vi "ConnectionClosed.vi"(6 "FinaErrorCode":i32, 8 "error in (no error)":errorcluster, 9 "ClientIP":string, 10 "ConnectionNumber":i32, 11 "TCP_Server in":refnum<class "TCP_Server.lvclass">) -> (0 "error out":errorcluster, 3 "TCP_Server out":refnum<class "TCP_Server.lvclass">)   [LabVIEW 2023, in "TCP_Server.lvlib" / "TCP_Server.lvclass"]
uses:
  TCP_Server.lvclass
  TCP_Server.lvclass/TCP_Server.ctl
  <vilib>/ActorFramework/Stop Msg/Stop Msg.lvclass
  76787049-4297-4f56-aecd-24274861dc6b.vi
  <vilib>/ActorFramework/Message Enqueuer/Message Enqueuer.lvclass
  TCP_Listener/TypeDefinitions/ConnectionInformation.ctl
  TCP_Listener/TCP_Listener.lvlib
  TypeDeclarations/ServerConnection.ctl
  TCP_Server.lvlib
  TCP_serverGUI/TCP_serverGUI Messages/UpdateConnectionsListbox Msg/UpdateConnectionsListbox Msg.lvclass
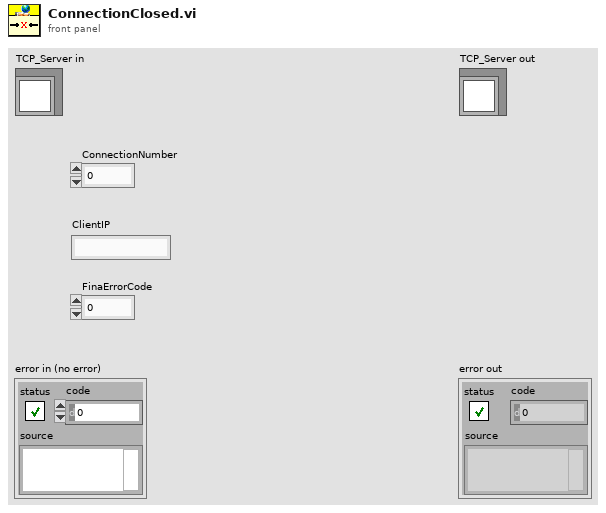
[diagram p1: front panel]
types:
  T1 = typedef "TCP_Server.lvlib/ServerConnection.ctl" = cluster{"Connection Handlers's Enqueuer":refnum<class "Message Enqueuer.lvclass">, "Connection Window's Enqueuer":refnum<class "Message Enqueuer.lvclass">, "Connection Information":T2}
  T2 = typedef "TCP_Listener.lvlib/ConnectionInformation.ctl" = cluster{"Connection number":i32, "Remote Address":string, "Remote Port":u16, "Connection ID":refnum<k5>}
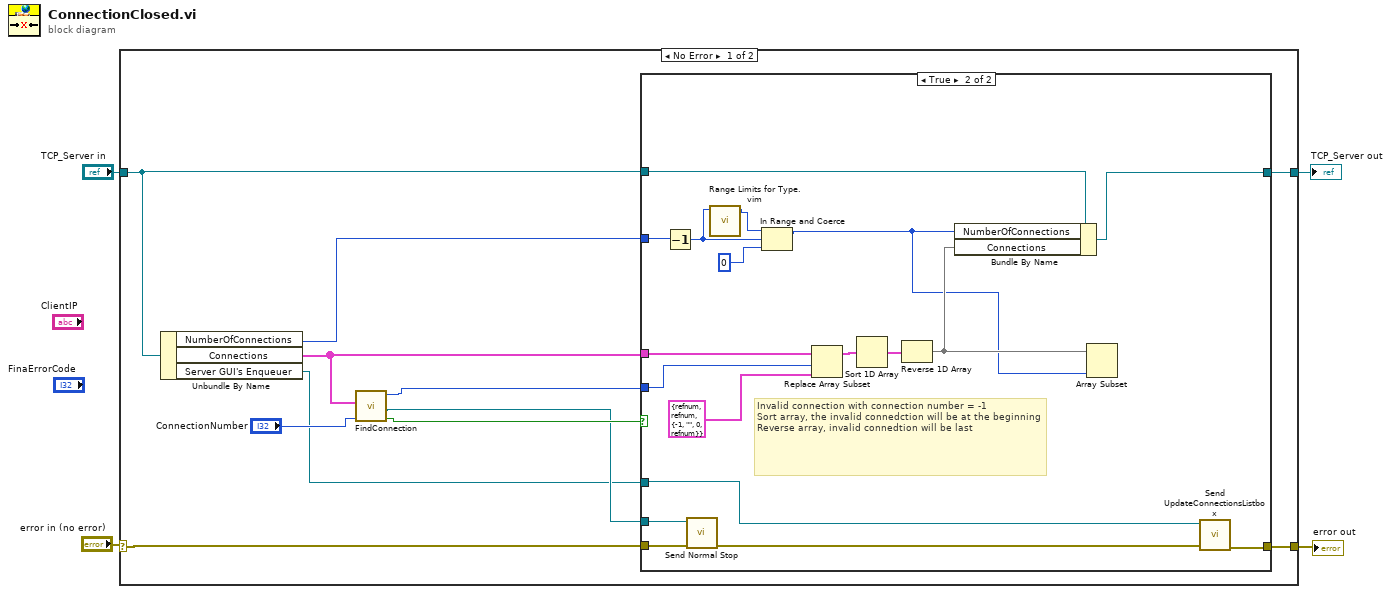
[diagram p0: block diagram]
diagram:
  n1 = case shown="No Error" "error in (no error)" {
    selector: "error in (no error)" -> [w12 w37]
    tunnel: [w11 w37] -> w3
    tunnel: "TCP_Server in" -> [w14 w36]
    tunnel: [w13 w36] -> w1
    frame No Error {
      n2 = Unbundle By Name(w14) -> ("NumberOfConnections"=w15:i32, "Connections"=w10:T1[], "Server GUI's Enqueuer"=w5:refnum<class "Message Enqueuer.lvclass">)
      n3 = call "FindConnection.vi"("Connection number"="ConnectionNumber", "Connections"=w10) -> ("Found?"=w8:bool, "Connection Window's Enqueuer"=w7:refnum<class "Message Enqueuer.lvclass">, "Connection index"=w9:i32)  [unwired: 6 in, 1 out]
      n4 = case shown="True" w8 {
        tunnel: w10 -> [_ w32]
        tunnel: w9 -> [_ w33]
        tunnel: w15 -> [_ w31]
        tunnel: w14 -> [w16 w30]
        tunnel: [w16 w29] -> w13
        tunnel: w12 -> [w17 w28]
        tunnel: [w17 w21] -> w11
        tunnel: w7 -> [_ w27]
        tunnel: w5 -> [_ w20]
        frame False {
        }
        frame True {
          # "Invalid connection with connection number = -1\nSort array, the invalid connedction will be at the beginning\nReverse array, invalid connedtion will be last"
          n5 = Decrement(x=w31) -> (x-1=w25:i32)
          n6 = call <vilib>:"Send Normal Stop.vi"("error in (no error)"=w28, "Message Enqueuer"=w27) -> ("error out"=w22:errorcluster)  [unwired: 9 in]
          n7 = call "Range Limits for Type.vim"("type"=w25) -> ("maximum value for type"=w24:i32)  [unwired: 9 in, 1 out]
          n8 = In Range and Coerce(upper limit=w24, x=w25, lower limit=0) -> (coerced(x)=w18:i32)  [unwired: 1 out]
          n9 = Replace Array Subset(array=w32, new element=T1 {"Connection Handlers's Enqueuer"=refnum, "Connection Window's Enqueuer"=refnum, "Connection Information"={"Connection number"=-1, "Remote Address"="", "Remote Port"=0, "Connection ID"=refnum}} ("new element/subarray"), index=w33) -> (w35:T1[])
          n10 = Sort 1D Array(array=w35) -> (sorted array=w34:T1[])
          n11 = Reverse 1D Array(array=w34) -> (reversed array=w19:T1[])
          n12 = Bundle By Name(cluster=w30, "NumberOfConnections"=w18, "Connections"=w19) -> (w29:refnum<class "TCP_Server.lvclass">)
          n13 = Array Subset(array=w19, length=w18) -> ()  [unwired: 1 in, 1 out]
          n14 = call "Send UpdateConnectionsListbox.vi"("error in (no error)"=w22, "Message Enqueuer"=w20) -> ("error out"=w21:errorcluster)  [unwired: 8 in, 1 out]
        }
      }
    }
    frame Error {
    }
  }
  "error out" <- w3
  "TCP_Server out" <- w1
